vi "Read.vi"   [LabVIEW 2024, in "Keithley 2450.lvlib"]
doc: "Allows users to read one or more measurements from the DMM."
uses:
  Keithley 2450.lvlib
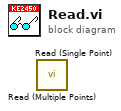
[diagram p0: block diagram]
diagram:
  n1 = call "Read (Multiple Points).vi"() -> ()  [unwired: 13 in, 3 out]
  n2 = call "Read (Single Point).vi"() -> ()  [unwired: 13 in, 3 out]
